vi "SetIIR.vi"(7 "filter":u8, 8 "error in (no error)":errorcluster, 11 "BME680 in":refnum<class "BME680.lvclass">) -> (0 "error out":errorcluster, 3 "BME680 out":refnum<class "BME680.lvclass">)   [LabVIEW 2022 SP3, in "BME680.lvlib" / "BME680.lvclass"]
uses:
  BME680.lvclass
  BME680.lvclass/BME680.ctl
  Typedefs/Conf.ctl
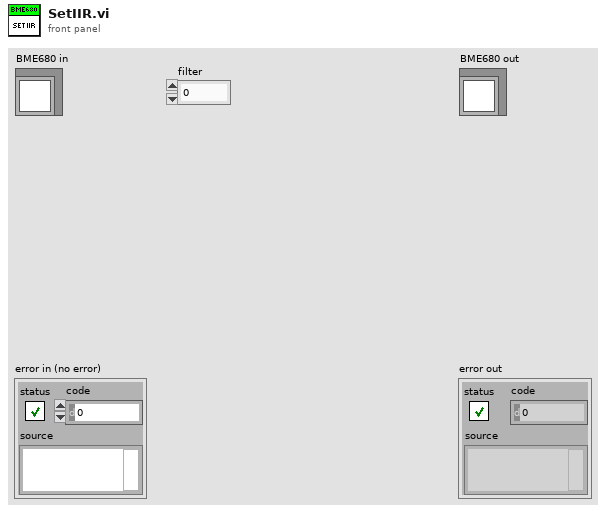
[diagram p1: front panel]
types:
  T1 = typedef "BME680.lvlib/BME680.lvclass/Conf.ctl" = cluster{"os_hum":u8, "os_temp":u8, "os_pres":u8, "filter":u8, "odr":u8}
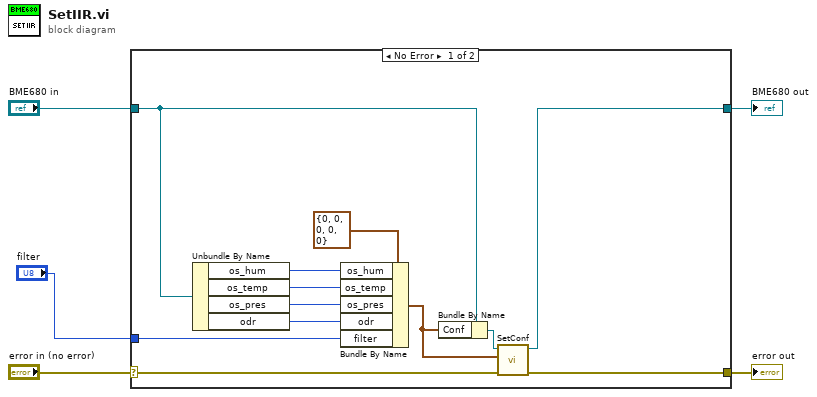
[diagram p0: block diagram]
diagram:
  n1 = case shown="No Error" "error in (no error)" {
    selector: "error in (no error)" -> [w17 w19]
    tunnel: [w16 w19] -> w4
    tunnel: [w15 w18] -> w2
    tunnel: "BME680 in" -> [w8 w18]
    tunnel: "filter" -> [w9 _]
    frame No Error {
      n2 = Unbundle By Name(w8) -> ("os_hum"=w13:u8, "os_temp"=w12:u8, "os_pres"=w11:u8, "odr"=w10:u8)
      n3 = Bundle By Name(cluster=T1 {"os_hum"=0, "os_temp"=0, "os_pres"=0, "filter"=0, "odr"=0} ("Conf"), "os_hum"=w13, "os_temp"=w12, "os_pres"=w11, "odr"=w10, "filter"=w9) -> (w6:T1)
      n4 = Bundle By Name(cluster=w8, "Conf"=w6) -> (w7:refnum<class "BME680.lvclass">)
      n5 = call-dynamic "SetConf.vi"("error in (no error)"=w17, "Conf"=w6, "BME68x in"=w7) -> ("error out"=w16:errorcluster, "BME68x out"=w15:refnum<class "BME680.lvclass">)  [unwired: 7 in]
    }
    frame Error {
    }
  }
  "error out" <- w4
  "BME680 out" <- w2
